vi "Time delay (SubVI).vi"(6 "Delay Time":dbl, 9 "input":dbl) -> (1 "Output":dbl)   [LabVIEW 2016]
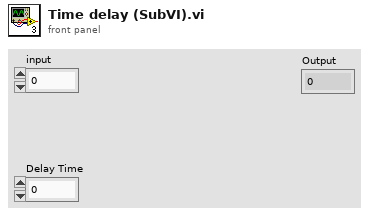
[diagram p1: front panel]
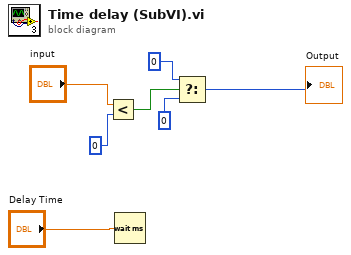
[diagram p0: block diagram]
diagram:
  n1 = Less?(x="input", y=0) -> (x < y?=w4:bool)
  n2 = Wait (ms)(milliseconds to wait="Delay Time") -> ()  [unwired: 1 out]
  n3 = Select(t=0, s=w4, f=0) -> (s? t:f=→"Output":i32)
